vi "Zstack acquisition with modified signal input_final_3color.vi"() -> ()   [LabVIEW 2020]
uses:
  <vilib>/DAQmx/write.llb/DAQmx Write (Digital 1D Bool 1Chan 1Samp).vi
  <vilib>/DAQmx/write.llb/DAQmx Write (Analog 1D Wfm NChan NSamp).vi
  <vilib>/Analysis/polynomials.llb/Polynomial Plot (Range).vi
  <vilib>/Utility/file.llb/Read Delimited Spreadsheet (DBL).vi
  <vilib>/DAQmx/create/channels.llb/DAQmx Create Channel (AO-Voltage-Basic).vi
  <vilib>/DAQmx/create/channels.llb/DAQmx Create Channel (CO-Pulse Generation-Ticks).vi
  <vilib>/DAQmx/configure/timing.llb/DAQmx Timing (Sample Clock).vi
  <vilib>/DAQmx/configure/timing.llb/DAQmx Timing (Implicit).vi
  <vilib>/DAQmx/create/channels.llb/DAQmx Create Channel (DO-Digital Output).vi
  <vilib>/DAQmx/miscellaneous.llb/DAQmx Fill In Error Info.vi
  <vilib>/DAQmx/create/channels.llb/DAQmx Create Channel (CO-Pulse Generation-Frequency).vi
  <vilib>/Analysis/NI_AALPro.lvlib
  <resource>/objmgr/daqmx.rc
  <vilib>/measure/NI_MABase.lvlib
panel:
  out "number of samples written per channel":u32=1
  in  "Stop":bool
  out "LabVIEW generated Sawtooth input (blue) and Camera trigger (red)":waveform(dbl)[](graph)=[{"t0"=timestamp(0 s since 1904-01-01), "dt"=1.0, "Y"=array[3075 elements]}, {"t0"=timestamp(0 s since 1904-01-01), "dt"=0.001, "Y"=array[3075 elements]}, {"t0"=timestamp(0 s since 1904-01-01), "dt"=0.001, "Y"=array[3075 elements]}, {"t0"=timestamp(0 s since 1904-01-01), "dt"=0.001, "Y"=array[3075 elements]}]
  in  "stop 2":bool caption="stop"
  out "# Samples written per channel":u32=3075
  out "actual frequency":dbl=1000.0
  in  "stop":bool
  in  "File to read":path=path "C:/Users/Hannah/Downloads/newcalibration_voice coil input_25msflyback_3075datapoints.txt"
  in  "P(x)":dbl[](array[numeric])=[-0.285, 0.654, -0.163]
  out "polynomial plot":cluster{dbl[], "P(A)":dbl[]}(graph)
  out "Signal input to voice coil (blue)":dbl[](graph)=[-0.285, -0.284345508671835, -0.2836913439966493, -0.2830375059744429, -0.2823839946052158, -0.28173080988896804, -0.28107795182569956, -0.28042542041541035, -0.27977321565810054, -0.27912133755376994, -0.27846978610241874, -0.27781856130404675, -0.2771676631586541, -0.2765170916662408, -0.2758668468268068, -0.275216928640352, -0.27456733710687664, -0.27391807222638054, -0.2732691339988637, -0.2726205224243262, -0.271972237502768, -0.2713242792341891, -0.27067664761858956, -0.27002934265596923, -0.2693823643463283, -0.2687357126896666, -0.2680893876859843, -0.2674433893352812, -0.26679771763755744, -0.266152372592813, -0.2655073542010479, -0.26486266246226203, -0.2642182973764555, -0.2635742589436283, -0.2629305471637804, -0.26228716203691177, -0.2616441035630225, -0.26100137174211246, -0.2603589665741818, -0.2597168880592304, -0.2590751361972583, -0.2584337109882655, -0.25779261243225204, -0.25715184052921786, -0.256511395279163, -0.2558712766820875, -0.25523148473799123, -0.25459201944687426, -0.2539528808087366, -0.2533140688235783, -0.2526755834913993, -0.25203742481219954, -0.2513995927859791, -0.25076208741273803, -0.2501249086924762, -0.24948805662519374, -0.24885153121089054, -0.24821533244956667, -0.24757946034122208, -0.2469439148858568, -0.24630869608347083, -0.24567380393406418, -0.2450392384376368, -0.24440499959418877, -0.24377108740372, -0.24313750186623057, -0.24250424298172044, -0.2418713107501896, -0.2412387051716381, -0.24060642624606587, -0.23997447397347293, -0.23934284835385933, -0.23871154938722505, -0.23808057707357003, -0.23744993141289436, -0.23681961240519797, -0.2361896200504809, -0.2355599543487431, -0.23493061529998463, -0.23430160290420549, -0.23367291716140562, -0.23304455807158508, -0.23241652563474383, -0.23178881985088187, -0.23116144071999925, -0.23053438824209593, -0.2299076624171719, -0.22928126324522718, -0.22865519072626178, -0.22802944486027565, -0.22740402564726886, -0.22677893308724137, -0.22615416718019318, -0.2255297279261243, -0.22490561532503472, -0.22428182937692445, -0.22365837008179348, -0.22303523743964182, -0.22241243145046946, -0.2217899521142764, -0.22116779943106268, -0.2205459734008282, -0.21992447402357307, -0.21930330129929726, -0.21868245522800073, -0.21806193580968353, -0.2174417430443456, -0.216821876931987, -0.2162023374726077, -0.21558312466620771, -0.21496423851278704, -0.21434567901234564, -0.2137274461648836, -0.2131095399704008, -0.21249196042889734, -0.21187470754037319, -0.2112577813048283, -0.21064118172226276, -0.21002490879267655, -0.2094089625160696, -0.20879334289244195, -0.20817804992179365, -0.20756308360412462, -0.2069484439394349, -0.2063341309277245, -0.20572014456899337, -0.20510648486324162, -0.20449315181046912, -0.20388014541067592, -0.20326746566386203, -0.20265511257002744, -0.2020430861291722, -0.20143138634129623, -0.20082001320639958, -0.2002089667244822, -0.19959824689554417, -0.19898785371958544, -0.19837778719660598, -0.19776804732660586, -0.19715863410958503, -0.19654954754554352, -0.1959407876344813, -0.1953323543763984, -0.1947242477712948, -0.19411646781917047, -0.1935090145200255, -0.1929018878738598, -0.19229508788067345, -0.19168861454046637, -0.19108246785323857, -0.19047664781899015, -0.18987115443772096, -0.18926598770943112, -0.18866114763412056, -0.18805663421178936, -0.1874524474424374, -0.1868485873260648, -0.18624505386267143, -0.18564184705225745, -0.18503896689482274, -0.18443641339036732, -0.18383418653889122, -0.1832322863403944, -0.18263071279487691, -0.18202946590233876, -0.18142854566277988, -0.18082795207620028, -0.1802276851426, -0.17962774486197908, -0.17902813123433742, -0.17842884425967506, -0.17782988393799204, -0.17723125026928827, -0.17663294325356382, -0.1760349628908187, -0.1754373091810529, -0.17483998212426638, -0.17424298172045916, -0.17364630796963126, -0.17304996087178265, -0.17245394042691337, -0.1718582466350234, -0.1712628794961127, -0.17066783901018132, -0.17007312517722922, -0.1694787379972565, -0.16888467747026303, -0.16829094359624888, -0.167697536375214, -0.1671044558071585, -0.16651170189208225, -0.1659192746299853, -0.1653271740208677, -0.16473540006472936, -0.16414395276157034, -0.16355283211139066, -0.16296203811419024, -0.16237157076996914, -0.16178143007872733, -0.16119161604046486, -0.1606021286551817, -0.16001296792287784, -0.15942413384355322, -0.15883562641720797, -0.15824744564384202, -0.15765959152345535, -0.157072064056048, -0.15648486324161998, -0.15589798908017125, -0.1553114415717018, -0.15472522071621167, -0.15413932651370088, -0.15355375896416934, -0.15296851806761713, -0.15238360382404423, -0.15179901623345066, -0.15121475529583633, -0.15063082101120134, -0.15004721337954569, -0.1494639324008693, -0.14888097807517225, -0.14829835040245445, -0.14771604938271604, -0.14713407501595688, -0.14655242730217702, -0.1459711062413765, -0.14539011183355524, -0.14480944407871332, -0.1442291029768507, -0.1436490885279674, -0.14306940073206337, -0.14249003958913864, -0.14191100509919327, -0.14133229726222715, -0.1407539160782404, -0.14017586154723288, -0.1395981336692047, -0.13902073244415583, -0.13844365787208626, -0.13786690995299603, -0.13729048868688504, -0.1367143940737534, -0.13613862611360106, -0.13556318480642804, -0.1349880701522343, -0.13441328215101986, -0.13383882080278475, -0.1332646861075289, -0.1326908780652524, -0.1321173966759552, -0.1315442419396373, -0.1309714138562987, -0.13039891242593943, -0.12982673764855943, -0.12925488952415876, -0.1286833680527374, -0.12811217323429533, -0.12754130506883257, -0.12697076355634912, -0.12640054869684497, -0.1258306604903201, -0.1252610989367746, -0.12469186403620838, -0.12412295578862143, -0.12355437419401383, -0.12298611925238548, -0.12241819096373646, -0.1218505893280668, -0.12128331434537637, -0.1207163660156653, -0.1201497443389335, -0.119583449315181, -0.11901748094440787, -0.11845183922661395, -0.11788652416179943, -0.11732153574996412, -0.1167568739911082, -0.11619253888523154, -0.11562853043233423, -0.11506484863241617, -0.11450149348547742, -0.11393846499151802, -0.11337576315053788, -0.11281338796253709, -0.11225133942751558, -0.11168961754547335, -0.11112822231641048, -0.11056715374032686, -0.1100064118172226, -0.10944599654709763, -0.10888590792995195, -0.10832614596578558, -0.10776671065459853, -0.10720760199639076, -0.1066488199911623, -0.10609036463891316, -0.10553223593964331, -0.10497443389335279, -0.10441695850004157, -0.10385980975970963, -0.10330298767235702, -0.10274649223798371, -0.10219032345658968, -0.10163448132817499, -0.1010789658527396, -0.1005237770302835, -0.09996891486080672, -0.09941437934430924, -0.09886017048079107, -0.0983062882702522, -0.09775273271269264, -0.0971995038081124, -0.09664660155651142, -0.0960940259578898, -0.09554177701224745, -0.0949898547195844, -0.09443825907990072, -0.09388699009319626, -0.09333604775947113, -0.09278543207872533, -0.09223514305095881, -0.09168518067617165, -0.09113554495436374, -0.09058623588553519, -0.09003725346968586, -0.08948859770681591, -0.08894026859692525, -0.08839226614001383, -0.0878445903360818, -0.08729724118512902, -0.0867502186871556, -0.08620352284216146, -0.08565715365014659, -0.08511111111111108, -0.08456539522505482, -0.08402000599197795, -0.08347494341188033, -0.08293020748476201, -0.082385798210623, -0.08184171558946332, -0.08129795962128292, -0.08075453030608179, -0.08021142764386005, -0.07966865163461759, -0.0791262022783544, -0.07858407957507055, -0.07804228352476594, -0.07750081412744073, -0.07695967138309479, -0.07641885529172815, -0.07587836585334079, -0.07533820306793276, -0.07479836693550404, -0.07425885745605462, -0.07371967462958451, -0.0731808184560937, -0.0726422889355822, -0.07210408606805, -0.07156620985349715, -0.0710286602919235, -0.07049143738332925, -0.06995454112771426, -0.06941797152507859, -0.06888172857542227, -0.06834581227874517, -0.0678102226350474, -0.06727495964432897, -0.06674002330658982, -0.06620541362183, -0.06567113059004948, -0.06513717421124829, -0.06460354448542632, -0.06407024141258374, -0.06353726499272042, -0.06300461522583639, -0.062472292111931726, -0.06194029565100631, -0.061408625843060255, -0.06087728268809345, -0.060346266186105973, -0.05981557633709783, -0.05928521314106894, -0.05875517659801943, -0.05822546670794915, -0.05769608347085822, -0.057167026886746575, -0.05663829695561426, -0.05610989367746122, -0.05558181705228746, -0.05505406708009308, -0.05452664376087796, -0.053999547094642164, -0.053472777081385675, -0.052946333721108435, -0.05242021701381058, -0.05189442695949201, -0.05136896355815271, -0.05084382680979274, -0.05031901671441208, -0.04979453327201072, -0.04927037648258867, -0.04874654634614592, -0.048223042862682475, -0.047699866032198335, -0.0471770158546935, -0.04665449233016797, -0.04613229545862174, -0.04561042524005482, -0.04508888167446723, -0.044567664761858916, -0.044046774502229935, -0.04352621089558023, -0.04300597394190983, -0.04248606364121876, -0.04196647999350697, -0.04144722299877451, -0.04092829265702133, -0.04040968896824751, -0.039891411932452936, -0.03937346154963772, -0.03885583781980173, -0.0383385407429451, -0.0378215703190678, -0.03730492654816975, -0.03678860943025106, -0.036272618965311615, -0.035756955153351505, -0.03524161799437073, -0.0347266074883692, -0.03421192363534703, -0.03369756643530414, -0.03318353588824058, -0.03266983199415624, -0.032156454753051344, -0.03164340416492567, -0.031130680229779273, -0.030618282947612263, -0.030106212318424475, -0.029594468342216074, -0.02908305101898695, -0.028571960348737047, -0.028061196331466587, -0.027550758967175293, -0.027040648255863442, -0.026530864197530812, -0.026021406792177515, -0.02551227603980355, -0.02500347194040886, -0.02449499449399345, -0.02398684370055737, -0.023479019560100622, -0.02297152207262315, -0.022464351238125013, -0.021957507056606096, -0.021450989528066566, -0.020944798652506313, -0.020438934429925393, -0.01993339686032375, -0.019428185943701437, -0.018923301680058457, -0.0184187440693947, -0.01791451311171033, -0.01741060880700518, -0.01690703115527936, -0.016403780156532932, -0.01590085581076567, -0.015398258117977848, -0.014895987078169193, -0.014394042691339926, -0.01389242495748999, -0.013391133876619332, -0.012890169448728006, -0.012389531673815901, -0.011889220551883184, -0.011389236082929743, -0.01088957826695558, -0.010390247103960804, -0.009891242593945249, -0.009392564736909081, -0.008894213532852135, -0.008396188981774577, -0.00789849108367624, -0.007401119838557235, -0.0069040752464175625, -0.006407357307257167, -0.005910966021076103, -0.005414901387874316, -0.004919163407651805, -0.004423752080408738, -0.003928667406144837, -0.003433909384860323, -0.002939478016555086, -0.0024453733012291257, -0.0019515952388824975, -0.0014581438295152016, -0.0009650190731271269, -0.00047222096971838434, 2.0250480710970464e-05, 0.0005123952781611041, 0.00100421342263185, 0.0014957049141233747, 0.0019868697526356227, 0.0024777079381684275, 0.002968219470722011, 0.0034584043502962625, 0.003948262576891293, 0.00443779415050688, 0.004926999071143245, 0.005415877338800279, 0.00590442895347798, 0.006392653915176516, 0.0068805522238956085, 0.007368123879635424, 0.007855368882395908, 0.008342287232177115, 0.0088288789289791, 0.009315143972801698, 0.009801082363644964, 0.010286694101508898, 0.01077197918639361, 0.01125693761829899, 0.011741569397225093, 0.012225874523171809, 0.012709852996139304, 0.013193504816127466, 0.013676829983136352, 0.014159828497165905, 0.01464250035821607, 0.015124845566287015, 0.015606864121378683, 0.01608855602349102, 0.016569921272624022, 0.017050959868777693, 0.017531671811952143, 0.018012057102147205, 0.018492115739363046, 0.0189718477235995, 0.019451253054856676, 0.019930331733134576, 0.02040908375843309, 0.020887509130752435, 0.02136560785009234, 0.02184337991645302, 0.02232082532983437, 0.02279794409023639, 0.023274736197659185, 0.023751201652102594, 0.024227340453566726, 0.024703152602051526, 0.025178638097557104, 0.025653796940083295, 0.026128629129630154, 0.026603134666197792, 0.027077313549786042, 0.02755116578039507, 0.02802469135802471, 0.028497890282675076, 0.028970762554346163, 0.02944330817303792, 0.029915527138750453, 0.030387419451483544, 0.030858985111237414, 0.03133022411801195, 0.031801136471807157, 0.03227172217262314, 0.03274198122045974, 0.03321191361531706, 0.033681519357195044, 0.034150798446093755, 0.03461975088201319, 0.03508837666495329, 0.03555667579491412, 0.036024648271895554, 0.036492294095897715, 0.0369596132669206, 0.037426605784964206, 0.03789327165002848, 0.03835961086211337, 0.038825623421219035, 0.039291309327345425, 0.03975666858049248, 0.04022170118066015, 0.0406864071278486, 0.04115078642205772, 0.041614839063287556, 0.042078565051538064, 0.04254196438680924, 0.04300503706910114, 0.043467783098413704, 0.043930202474747104, 0.04439229519810106, 0.04485406126847569, 0.04531550068587109, 0.04577661345028711, 0.04623739956172396, 0.046697859020181365, 0.04715799182565955, 0.047617797978158405, 0.04807727747767787, 0.04853643032421817, 0.048995256517779084, 0.04945375605836072, 0.04991192894596297, 0.050369775180585996, 0.0508272947622298, 0.05128448769089411, 0.05174135396657925, 0.05219789358928495, 0.05265410655901154, 0.05310999287575868, 0.05356555253952655, 0.05402078555031514, 0.054475691908124346, 0.054930271612954384, 0.05538452466480498, 0.05583845106367635, 0.05629205080956834, 0.05674532390248105, 0.05719827034241459, 0.05765089012936864, 0.05810318326334346, 0.05855514974433895, 0.05900678957235517, 0.05945810274739205, 0.059909089269449656, 0.060359749138527985, 0.060810082354626926, 0.06126008891774659, 0.06170976882788698, 0.06215912208504809, 0.06260814868922976, 0.06305684864043226, 0.06350522193865543, 0.06395326858389927, 0.06440098857616383, 0.064848381915449, 0.06529544860175496, 0.06574218863508158, 0.06618860201542892, 0.06663468874279693, 0.06708044881718556, 0.06752588223859501, 0.06797098900702508, 0.06841576912247588, 0.06886022258494734, 0.06930434939443952, 0.06974814955095238, 0.0701916230544859, 0.07063476990504025, 0.07107759010261516, 0.0715200836472108, 0.07196225053882715, 0.07240409077746413, 0.07284560436312199, 0.07328679129580035, 0.07372765157549949, 0.0741681852022193, 0.07460839217595977, 0.07504827249672097, 0.07548782616450289, 0.07592705317930548, 0.07636595354112874, 0.07680452724997272, 0.07724277430583737, 0.0776806947087228, 0.07811828845862884, 0.07855555555555555, 0.07899249599950303, 0.07942910979047119, 0.07986539692846006, 0.08030135741346961, 0.08073699124549977, 0.0811722984245507, 0.08160727895062231, 0.08204193282371469, 0.08247626004382763, 0.08291026061096135, 0.08334393452511574, 0.08377728178629085, 0.08421030239448662, 0.08464299634970307, 0.08507536365194024, 0.08550740430119813, 0.08593911829747669, 0.08637050564077597, 0.08680156633109587, 0.08723230036843654, 0.08766270775279789, 0.08809278848417995, 0.08852254256258263, 0.08895196998800603, 0.08938107076045021, 0.089809844879915, 0.09023829234640052, 0.0906664131599067, 0.0910942073204336, 0.09152167482798113, 0.09194881568254948, 0.0923756298841385, 0.09280211743274808, 0.09322827832837849, 0.09365411257102946, 0.09407962016070132, 0.09450480109739373, 0.09492965538110687, 0.09535418301184073, 0.0957783839895952, 0.09620225831437051, 0.09662580598616638, 0.09704902700498302, 0.09747192137082028, 0.09789448908367826, 0.09831673014355707, 0.09873864455045639, 0.09916023230437648, 0.09958149340531725, 0.10000242785327873, 0.10042303564826088, 0.10084331679026376, 0.10126327127928736, 0.10168289911533157, 0.1021022002983965, 0.10252117482848216, 0.10293982270558855, 0.10335814392971548, 0.10377613850086326, 0.1041938064190317, 0.1046111476842208, 0.10502816229643064, 0.10544485025566108, 0.1058612115619123, 0.1062772462151842, 0.10669295421547681, 0.10710833556279009, 0.10752339025712399, 0.10793811829847871, 0.10835251968685405, 0.10876659442225012, 0.10918034250466685, 0.1095937639341043, 0.11000685871056248, 0.11041962683404127, 0.11083206830454084, 0.11124418312206102, 0.11165597128660193, 0.11206743279816361, 0.11247856765674591, 0.11288937586234893, 0.11329985741497256, 0.11371001231461697, 0.114119840561282, 0.11452934215496785, 0.11493851709567426, 0.11534736538340146, 0.11575588701814932, 0.11616408199991785, 0.11657195032870715, 0.11697949200451707, 0.11738670702734771, 0.11779359539719908, 0.11820015711407106, 0.11860639217796382, 0.11901230058887718, 0.11941788234681133, 0.11982313745176615, 0.12022806590374158, 0.12063266770273778, 0.12103694284875471, 0.12144089134179231, 0.12184451318185052, 0.12224780836892951, 0.12265077690302917, 0.12305341878414955, 0.12345573401229065, 0.12385772258745231, 0.12425938450963481, 0.12466071977883791, 0.1250617283950618, 0.12546241035830635, 0.12586276566857152, 0.12626279432585746, 0.12666249633016402, 0.12706187168149136, 0.1274609203798393, 0.12785964242520803, 0.12825803781759737, 0.1286561065570075, 0.12905384864343833, 0.12945126407688973, 0.1298483528573619, 0.1302451149848547, 0.13064155045936832, 0.1310376592809026, 0.1314334414494575, 0.13182889696503314, 0.13222402582762943, 0.1326188280372465, 0.1330133035938842, 0.1334074524975426, 0.13380127474822168, 0.13419477034592148, 0.13458793929064206, 0.1349807815823832, 0.1353732972211451, 0.13576548620692763, 0.136157348539731, 0.13654888421955497, 0.1369400932463996, 0.13733097562026497, 0.13772153134115095, 0.13811176040905782, 0.13850166282398518, 0.13889123858593333, 0.1392804876949021, 0.13966941015089163, 0.14005800595390194, 0.14044627510393282, 0.1408342176009844, 0.14122183344505668, 0.14160912263614966, 0.14199608517426343, 0.14238272105939775, 0.14276903029155286, 0.14315501287072857, 0.14354066879692506, 0.14392599807014222, 0.1443110006903801, 0.1446956766576386, 0.14508002597191788, 0.14546404863321782, 0.1458477446415385, 0.14623111399687982, 0.14661415669924177, 0.14699687274862455, 0.14737926214502794, 0.14776132488845206, 0.1481430609788969, 0.1485244704163623, 0.14890555320084853, 0.14928630933235543, 0.149666738810883, 0.15004684163643123, 0.15042661780900024, 0.15080606732858992, 0.15118519019520027, 0.15156398640883134, 0.15194245596948303, 0.1523205988771555, 0.15269841513184862, 0.15307590473356236, 0.153453067682297, 0.15382990397805213, 0.1542064136208281, 0.15458259661062473, 0.15495845294744193, 0.15533398263127995, 0.15570918566213865, 0.15608406204001807, 0.15645861176491815, 0.15683283483683885, 0.15720673125578033, 0.15758030102174247, 0.1579535441347254, 0.15832646059472888, 0.1586990504017532, 0.15907131355579807, 0.15944325005686372, 0.1598148599049501, 0.16018614310005702, 0.16055709964218473, 0.16092772953133316, 0.16129803276750232, 0.16166800935069214, 0.16203765928090252, 0.16240698255813374, 0.16277597918238562, 0.16314464915365823, 0.16351299247195145, 0.16388100913726544, 0.16424869914960005, 0.16461606250895544, 0.16498309921533155, 0.16534980926872822, 0.16571619266914567, 0.16608224941658378, 0.16644797951104262, 0.16681338295252218, 0.16717845974102236, 0.16754320987654325, 0.16790763335908487, 0.16827173018864716, 0.16863550036523012, 0.1689989438888338, 0.16936206075945814, 0.16972485097710327, 0.17008731454176906, 0.17044945145345547, 0.17081126171216265, 0.17117274531789045, 0.17153390227063908, 0.17189473257040833, 0.17225523621719824, 0.17261541321100887, 0.17297526355184012, 0.17333478723969226, 0.1736939842745649, 0.1740528546564583, 0.17441139838537234, 0.17476961546130715, 0.17512750588426274, 0.17548506965423888, 0.17584230677123575, 0.17619921723525328, 0.17655580104629154, 0.17691205820435063, 0.17726798870943017, 0.1776235925615306, 0.17797886976065153, 0.1783338203067933, 0.17868844419995572, 0.17904274144013888, 0.17939671202734264, 0.1797503559615672, 0.18010367324281246, 0.18045666387107834, 0.18080932784636494, 0.18116166516867216, 0.1815136758380002, 0.18186535985434893, 0.18221671721771826, 0.18256774792810837, 0.18291845198551904, 0.18326882938995054, 0.1836188801414027, 0.18396860423987554, 0.18431800168536905, 0.18466707247788333, 0.18501581661741828, 0.1853642341039739, 0.18571232493755024, 0.1860600891181472, 0.18640752664576493, 0.18675463752040333, 0.18710142174206246, 0.18744787931074225, 0.18779401022644265, 0.1881398144891639, 0.18848529209890574, 0.18883044305566837, 0.18917526735945162, 0.18951976501025553, 0.18986393600808021, 0.19020778035292546, 0.1905512980447916, 0.19089448908367834, 0.19123735346958576, 0.19157989120251384, 0.19192210228246265, 0.19226398670943223, 0.19260554448342238, 0.1929467756044333, 0.19328768007246488, 0.19362825788751714, 0.19396850904959018, 0.19430843355868382, 0.19464803141479825, 0.19498730261793323, 0.19532624716808905, 0.19566486506526554, 0.19600315630946263, 0.19634112090068057, 0.196678758838919, 0.19701607012417827, 0.1973530547564582, 0.19768971273575886, 0.19802604406208013, 0.19836204873542213, 0.19869772675578484, 0.19903307812316823, 0.1993681028375724, 0.1997028008989971, 0.2000371723074426, 0.20037121706290878, 0.20070493516539567, 0.20103832661490328, 0.20137139141143146, 0.20170412955498046, 0.20203654104555008, 0.20236862588314047, 0.20270038406775148, 0.20303181559938321, 0.20336292047803567, 0.20369369870370874, 0.20402415027640258, 0.2043542751961171, 0.20468407346285228, 0.20501354507660818, 0.2053426900373848, 0.2056715083451821, 0.20600000000000002]
  out "Error out":errorcluster
  in  "Disable Axis":bool
  in  "Z step size (um)":dbl=0.2
  out "Number of Slices":dbl=400.0
  in  "Input will be multiplied by 5":dbl=80.0
  in  "Acquire Z Stack?":bool=TRUE
  out "GetFirmwareVersion 2":string="3.03\r"
  out "Connected":bool=TRUE
  in  "SPIIPLUSCOM660Lib.IAsyncChannel":refnum<k7>
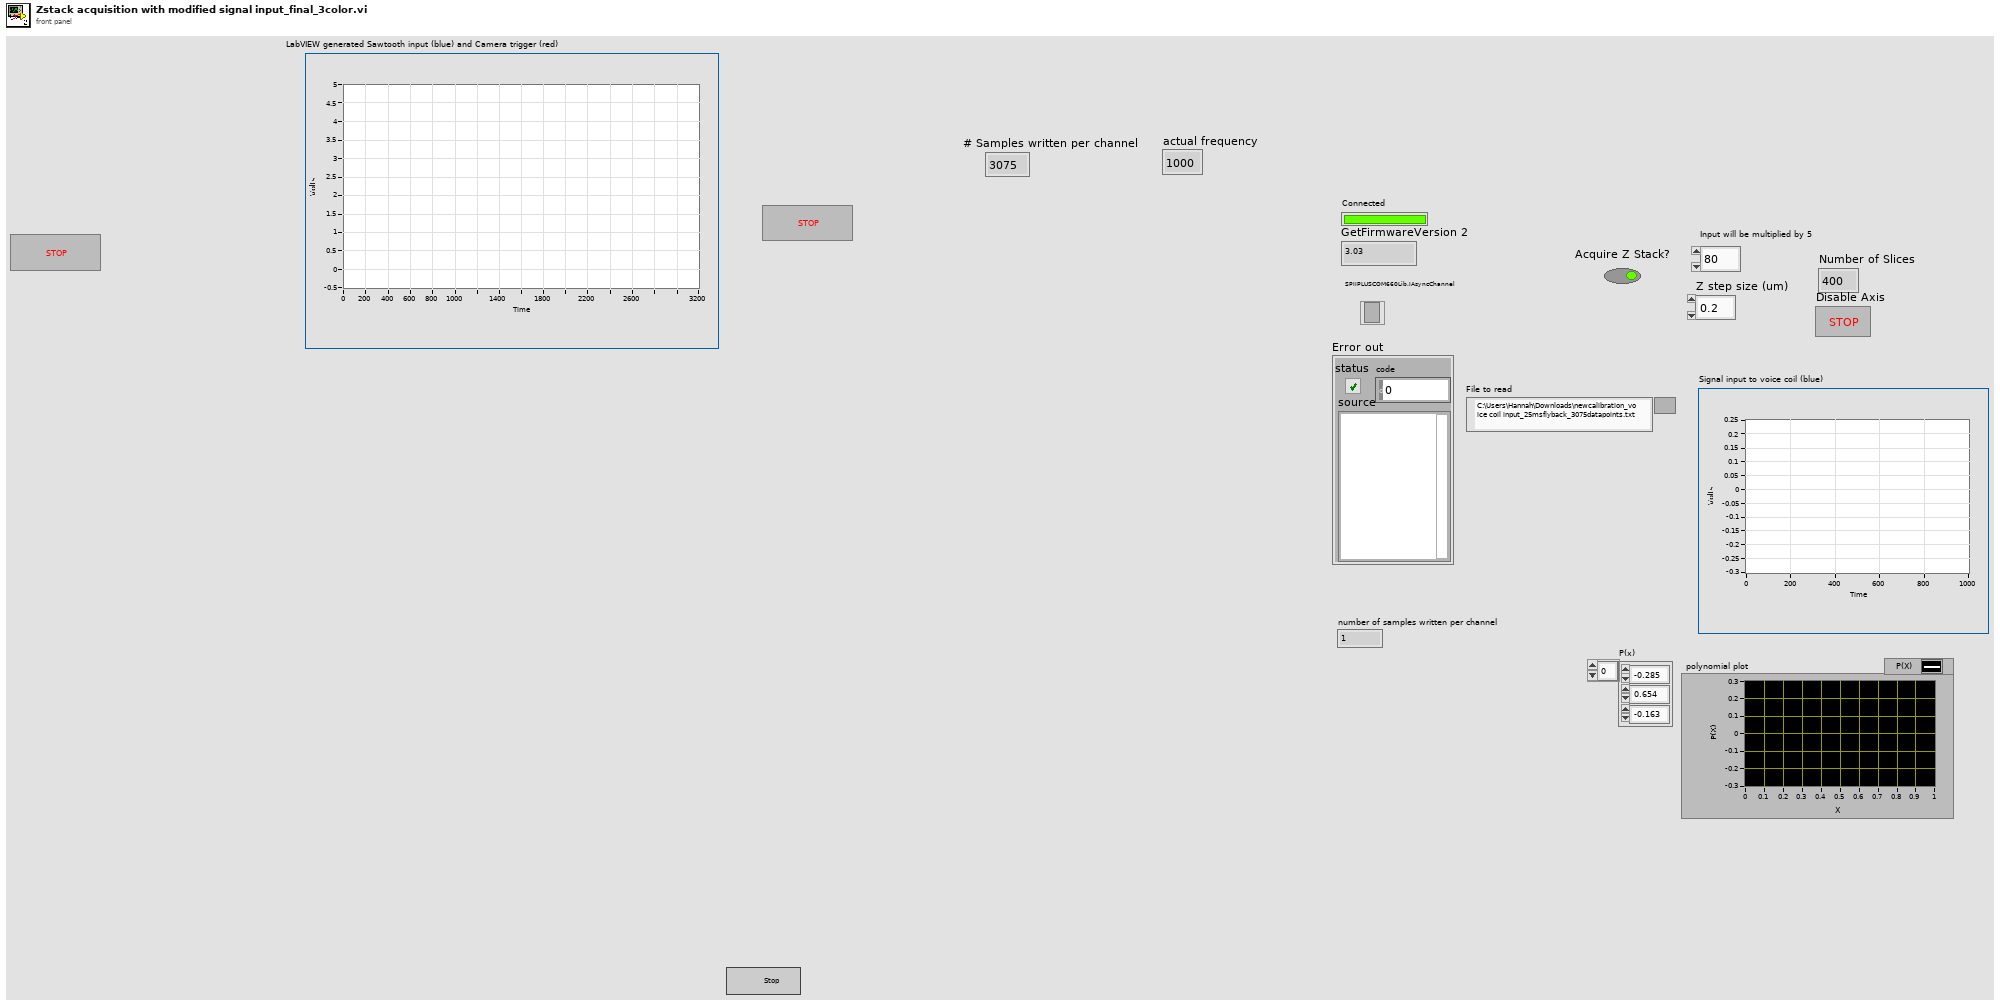
[diagram p1: front panel]
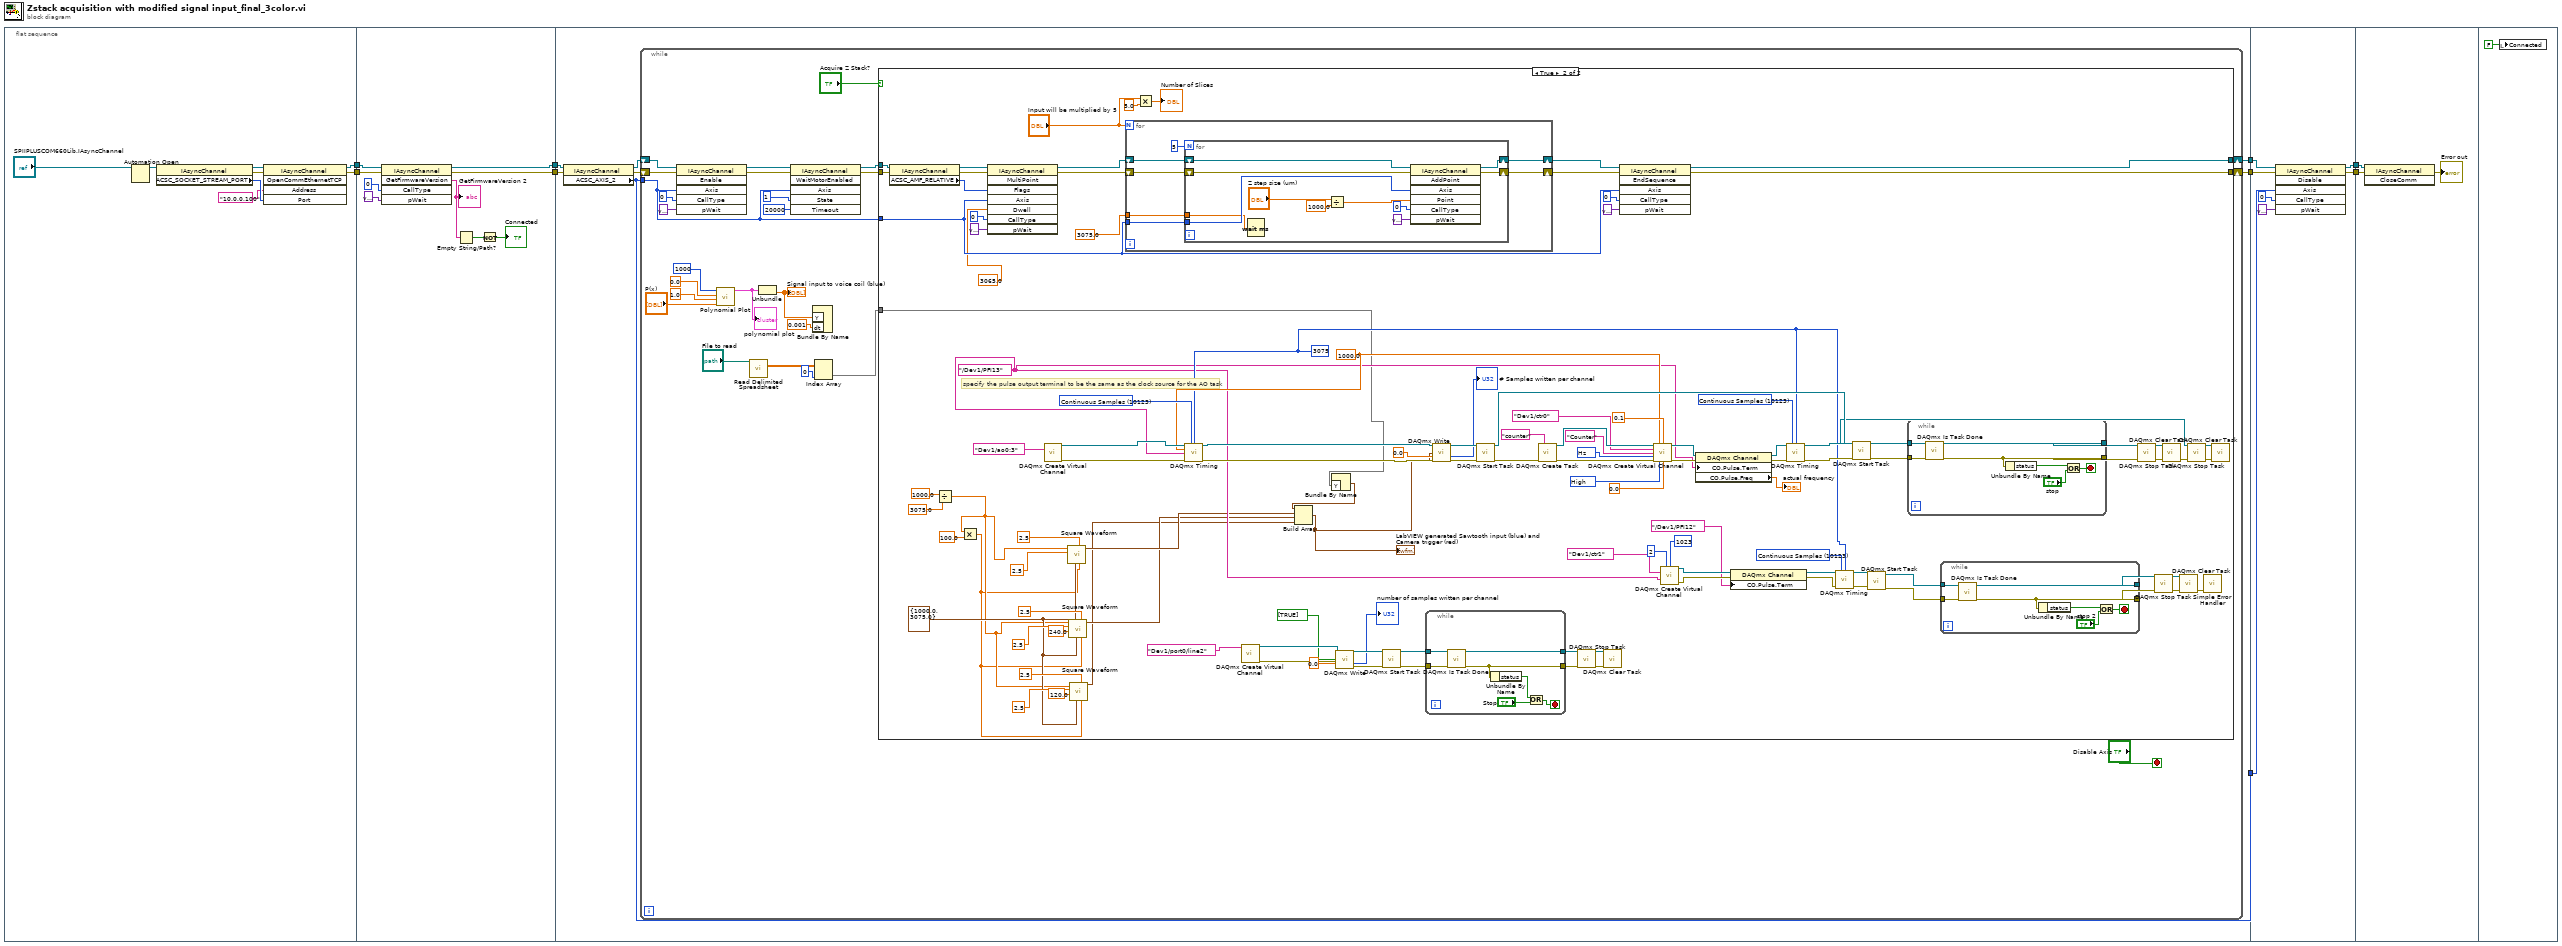
[diagram p0: block diagram]
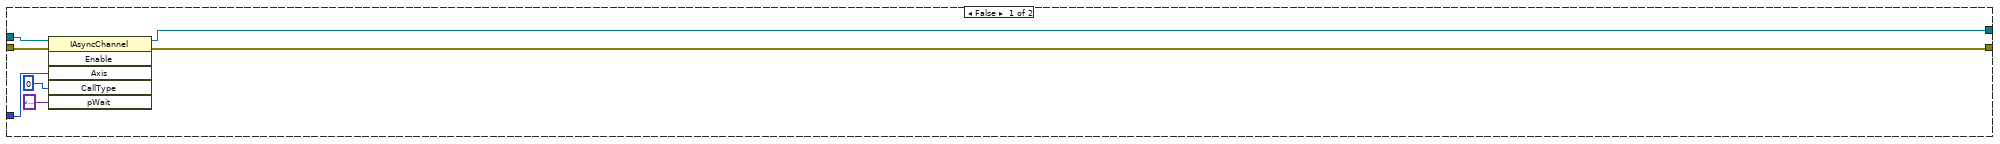
[diagram p2: hidden frame]
diagram:
  n1 = flat-sequence {
    tunnel: [w12] -> w9
    tunnel: [w11] -> w8
    tunnel: w9 -> [w22]
    tunnel: w8 -> [w21]
    tunnel: [w19] -> w7
    tunnel: [w18] -> w6
    tunnel: w7 -> [w31]
    tunnel: w6 -> [w30]
    tunnel: [w33] -> w5
    tunnel: [w32] -> w4
    tunnel: [w29] -> w3
    tunnel: w5 -> [w226]
    tunnel: w4 -> [w225]
    tunnel: [w224] -> w2
    tunnel: [w223] -> w1
    tunnel: w3 -> [w222]
    tunnel: w2 -> [w228]
    tunnel: w1 -> [w227]
    frame #0 {
      n2 = Automation Open(Automation Refnum="SPIIPLUSCOM660Lib.IAsyncChannel") -> (Automation Refnum=w17:refnum<k7>)  [unwired: 3 in, 1 out]
      n3 = property class="IAsyncChannel"(reference=w17) -> (reference out=w16:refnum<k7>, error out=w10:errorcluster, "ACSC_SOCKET_STREAM_PORT"=w14:i32)  [unwired: 1 in]
      n4 = invoke class="IAsyncChannel" method="OpenCommEthernetTCP"(reference=w16, error in=w10, "Address"="10.0.0.100", "Port"=w14) -> (reference out=w12:refnum<k7>, error out=w11:errorcluster)  [unwired: 1 in, 3 out]
    }
    frame #1 {
      n5 = invoke class="IAsyncChannel" method="GetFirmwareVersion"(reference=w22, error in=w21, "CallType"=u64 0, "pWait"=variant) -> (reference out=w19:refnum<k7>, error out=w18:errorcluster, "GetFirmwareVersion"=w24:string)  [unwired: 1 in, 2 out]
      "GetFirmwareVersion 2" <- w24
      n6 = Empty String/Path?(string/path=w24) -> (empty?=w23:bool)
      n7 = Not(x=w23) -> (.not. x?=→"Connected":bool)
    }
    frame #2 {
      n8 = property class="IAsyncChannel"(reference=w31, error in=w30) -> (reference out=w28:refnum<k7>, error out=w27:errorcluster, "ACSC_AXIS_2"=w29:i32)
      n9 = while {
        shift-right: [w59] -> w33
        shift-left: w28 -> [w51]
        shift-right: [w58] -> w32
        shift-left: w27 -> [w50]
        tunnel: w29 -> [w47]
        stop <- "Disable Axis" stop-if-true
        n10 = invoke class="IAsyncChannel" method="Enable"(reference=w51, error in=w50, "Axis"=w47, "CallType"=u64 0, "pWait"=variant) -> (reference out=w55:refnum<k7>, error out=w54:errorcluster)  [unwired: 1 in, 4 out]
        n11 = call-poly <vilib>:"Polynomial Plot.vi"("P(x)"="P(x)", "end"=1.0, "start"=0.0, "samples"=1000) -> ("polynomial plot"=w43:cluster{"Ramp Pattern":dbl[], "P(A)":dbl[]})  [unwired: 6 in, 1 out]
        "polynomial plot" <- w43
        n12 = call-poly <vilib>:"Read Delimited Spreadsheet.vi"("file path (dialog if empty)"="File to read") -> ("all rows"=w36:dbl[][])  [unwired: 9 in, 5 out]
        n13 = Unbundle(w43) -> ("P(A)"=w38:dbl[])  [unwired: 1 out]
        "Signal input to voice coil (blue)" <- w38
        n14 = invoke class="IAsyncChannel" method="WaitMotorEnabled"(reference=w55, error in=w54, "Axis"=w47, "State"=1, "Timeout"=20000) -> (reference out=w46:refnum<k7>, error out=w45:errorcluster)  [unwired: 1 in, 4 out]
        n15 = Bundle By Name("Y"=w38, "dt"=0.001) -> ()  [unwired: 1 in, 1 out]
        n16 = Index Array(array=w36, index (col)=0 ("disabled index (col)")) -> (element=w34:dbl[])  [unwired: 1 in]
        n17 = case shown="True" "Acquire Z Stack?" {
          tunnel: w46 -> [w66 w168]
          tunnel: w45 -> [w65 w169]
          tunnel: [w64 w166] -> w59
          tunnel: [w63 w167] -> w58
          tunnel: w47 -> [w62 w165]
          tunnel: w34 -> [_ w86]
          frame False {
            n18 = invoke class="IAsyncChannel" method="Enable"(reference=w66, error in=w65, "Axis"=w62, "CallType"=u64 0, "pWait"=variant) -> (reference out=w64:refnum<k7>, error out=w63:errorcluster)  [unwired: 1 in, 4 out]
          }
          frame True {
            w71 = cluster{"Fs":dbl, "#s":dbl} {"Fs"=1000.0, "#s"=3075.0} ("sampling info")
            w102 = 3075 ("samples per channel")
            w105 = 10123 items=["Finite Samples"=10178, "Continuous Samples"=10123, "Hardware Timed Single Point"=12522] ("sample mode")
            w131 = 10192 items=["High"=10192, "Low"=10214] ("idle state")
            w132 = 10373 items=["Hz"=10373] ("units")
            w101 = tag "/Dev1/PFI13" ("CO.Pulse.Term")
            w119 = 10123 items=["Finite Samples"=10178, "Continuous Samples"=10123, "Hardware Timed Single Point"=12522] ("sample mode")
            w115 = 1000.0 ("rate")
            w157 = 10123 items=["Finite Samples"=10178, "Continuous Samples"=10123, "Hardware Timed Single Point"=12522] ("sample mode")
            # "specify the pulse output terminal to be the same as the clock source for the AO task"
            n19 = property class="IAsyncChannel"(reference=w168, error in=w169) -> (reference out=w178:refnum<k7>, error out=w177:errorcluster, "ACSC_AMF_RELATIVE"=w174:i32)
            n20 = Divide(x=1000.0, y=3075.0) -> (x/y=w69:dbl)
            n21 = Multiply(x=w69, y=100.0) -> (x*y=w68:dbl)
            n22 = invoke class="IAsyncChannel" method="MultiPoint"(reference=w178, error in=w177, "Flags"=w174, "Axis"=w165, "Dwell"=3065.0, "CallType"=u64 0, "pWait"=variant) -> (reference out=w173:refnum<k7>, error out=w172:errorcluster)  [unwired: 1 in, 6 out]
            n23 = call-poly <vilib>:"DAQmx Create Virtual Channel.vi"("physical channels"=tag "Dev1/ao0:3") -> ("task out"=w159:refnum<k21>, "error out"=w158:errorcluster)  [unwired: 13 in]
            n24 = call <vilib>:"Square Waveform.vi"("duty cycle (%)"=w68, "offset"=2.5, "sampling info"=w71, "amplitude"=2.5 ("Amplitude for laser 1 (Max value 2.5)"), "frequency"=w69) -> ("signal out"=w99:waveform(dbl))  [unwired: 5 in, 1 out]
            n25 = call <vilib>:"Square Waveform.vi"("duty cycle (%)"=w68, "offset"=2.5, "sampling info"=w71, "phase"=240.0, "amplitude"=2.5 ("Amplitude for laser 1 (Max value 2.5)"), "frequency"=w69) -> ("signal out"=w95:waveform(dbl))  [unwired: 4 in, 1 out]
            n26 = call <vilib>:"Square Waveform.vi"("duty cycle (%)"=w68, "offset"=2.5, "sampling info"=w71, "phase"=120.0, "amplitude"=2.5 ("Amplitude for laser 1 (Max value 2.5)"), "frequency"=w69) -> ("signal out"=w92:waveform(dbl))  [unwired: 4 in, 1 out]
            n27 = for {
              N: "Input will be multiplied by 5" -> [_]
              tunnel: w165 -> [w204]
              tunnel: 3075.0 ("Dwell") -> [w203]
              shift-right: [w206] -> w171
              shift-left: w173 -> [w208]
              shift-right: [w205] -> w170
              shift-left: w172 -> [w207]
              n28 = for {
                N: 5 -> [_]
                tunnel: w204 -> [w219]
                shift-right: [w214] -> w206
                shift-left: w208 -> [w218]
                shift-right: [w213] -> w205
                shift-left: w207 -> [w217]
                tunnel: w203 -> [w209]
                n29 = Wait (ms)(milliseconds to wait=w209) -> ()  [unwired: 1 out]
                n30 = Divide(x="Z step size (um)", y=1000.0) -> (x/y=w210:dbl)
                n31 = invoke class="IAsyncChannel" method="AddPoint"(reference=w218, error in=w217, "Axis"=w219, "Point"=w210, "CallType"=u64 0, "pWait"=variant) -> (reference out=w214:refnum<k7>, error out=w213:errorcluster)  [unwired: 1 in, 5 out]
              }
            }
            n32 = Multiply(x="Input will be multiplied by 5", y=5.0) -> (x*y=→"Number of Slices":dbl)
            n33 = call-poly <vilib>:"DAQmx Timing.vi"("task/channels in"=w159, "sample mode"=w157, "samples per channel"=w102, "rate"=w115, "source"=w101, "error in"=w158) -> ("task out"=w124:refnum<k21>, "error out"=w123:errorcluster)  [unwired: 8 in]
            n34 = call-poly <vilib>:"DAQmx Create Virtual Channel.vi"("lines"=tag "Dev1/port0/line2") -> ("task out"=w85:refnum<k21>, "error out"=w84:errorcluster)  [unwired: 13 in]
            n35 = Bundle By Name("Y"=w86) -> (w88:waveform(dbl))  [unwired: 1 in]
            n36 = Build Array(w88, w99, w95, w92) -> (w87:waveform(dbl)[])
            "LabVIEW generated Sawtooth input (blue) and Camera trigger (red)" <- w87
            n37 = call-poly <vilib>:"DAQmx Write.vi"("task/channels in"=w85, "data"=bool[] [TRUE], "timeout"=0.0, "error in"=w84) -> ("task out"=w83:refnum<k21>, "number of samples written per channel"=→"number of samples written per channel":u32, "error out"=w82:errorcluster)  [unwired: 9 in]
            n38 = call <vilib>:"DAQmx Start Task.vi"("task/channels in"=w83, "error in"=w82) -> ("task out"=w81:refnum<k21>, "error out"=w80:errorcluster)  [unwired: 12 in]
            n39 = while {
              tunnel: w81 -> [w187]
              tunnel: w80 -> [w186]
              tunnel: [w184] -> w76
              tunnel: [w185] -> w77
              stop <- w181 stop-if-true
              n40 = call <vilib>:"DAQmx Is Task Done.vi"("task/channels in"=w187, "error in"=w186) -> ("task out"=w185:refnum<k21>, "error out"=w184:errorcluster)  [unwired: 11 in, 1 out]
              n41 = Unbundle By Name(w184) -> ("status"=w183:bool)
              n42 = Or(x=w183, y="Stop") -> (x .or. y?=w181:bool)
            }
            n43 = call-poly <vilib>:"DAQmx Write.vi"("task/channels in"=w124, "data"=w87, "timeout"=0.0, "error in"=w123) -> ("task out"=w137:refnum<k21>, "number of samples written per channel"=→"# Samples written per channel":u32, "error out"=w136:errorcluster)  [unwired: 9 in]
            n44 = call <vilib>:"DAQmx Start Task.vi"("task/channels in"=w137, "error in"=w136) -> ("task out"=w130:refnum<k21>, "error out"=w129:errorcluster)  [unwired: 12 in]
            n45 = call <vilib>:"DAQmx Create Task.vi"("new task name"="counter", "error in"=w129) -> ("task out"=w152:refnum<k21>, "error out"=w150:errorcluster)  [unwired: 12 in]
            n46 = call <vilib>:"DAQmx Stop Task.vi"("task/channels in"=w77, "error in"=w76) -> ("task out"=w79:refnum<k21>, "error out"=w78:errorcluster)  [unwired: 12 in]
            n47 = call <vilib>:"DAQmx Clear Task.vi"("task in"=w79, "error in"=w78) -> ()  [unwired: 13 in, 1 out]
            n48 = invoke class="IAsyncChannel" method="EndSequence"(reference=w171, error in=w170, "Axis"=w165, "CallType"=u64 0, "pWait"=variant) -> (reference out=w166:refnum<k7>, error out=w167:errorcluster)  [unwired: 1 in, 4 out]
            n49 = call-poly <vilib>:"DAQmx Create Virtual Channel.vi"("task in"=w152, "frequency"=w115, "duty cycle"=0.1, "counter"=tag "Dev1/ctr0", "name to assign"="Counter", "units"=w132, "error in"=w150, "idle state"=w131, "initial delay"=0.0) -> ("task out"=w149:refnum<k21>, "error out"=w148:errorcluster)  [unwired: 5 in]
            n50 = call-poly <vilib>:"DAQmx Create Virtual Channel.vi"("high ticks"=u32 2, "low ticks"=u32 1023, "counter"=tag "Dev1/ctr1", "source of ticks"=w101) -> ("task out"=w114:refnum<k21>, "error out"=w113:errorcluster)  [unwired: 10 in]
            n51 = property class="DAQmx Channel"(reference=w149, error in=w148, "CO.Pulse.Term"=w101) -> (reference out=w145:refnum<k21>, error out=w146:errorcluster, "CO.Pulse.Freq"=→"actual frequency":dbl)
            n52 = property class="DAQmx Channel"(reference=w114, error in=w113, "CO.Pulse.Term"=tag "/Dev1/PFI12") -> (reference out=w107:refnum<k21>, error out=w106:errorcluster)
            n53 = call-poly <vilib>:"DAQmx Timing.vi"("task/channels in"=w145, "sample mode"=w119, "samples per channel"=w102, "error in"=w146) -> ("task out"=w155:refnum<k21>, "error out"=w154:errorcluster)  [unwired: 10 in]
            n54 = call-poly <vilib>:"DAQmx Timing.vi"("task/channels in"=w107, "sample mode"=w105, "samples per channel"=w102, "error in"=w106) -> ("task out"=w104:refnum<k21>, "error out"=w103:errorcluster)  [unwired: 10 in]
            n55 = call <vilib>:"DAQmx Start Task.vi"("task/channels in"=w155, "error in"=w154) -> ("task out"=w126:refnum<k21>, "error out"=w138:errorcluster)  [unwired: 12 in]
            n56 = call <vilib>:"DAQmx Start Task.vi"("task/channels in"=w104, "error in"=w103) -> ("task out"=w111:refnum<k21>, "error out"=w110:errorcluster)  [unwired: 12 in]
            n57 = while {
              tunnel: w130 -> [w201]
              tunnel: w138 -> [w200]
              tunnel: [w199] -> w141
              tunnel: [w198] -> w142
              stop <- w195 stop-if-true
              n58 = call <vilib>:"DAQmx Is Task Done.vi"("task/channels in"=w201, "error in"=w200) -> ("task out"=w199:refnum<k21>, "error out"=w198:errorcluster)  [unwired: 11 in, 1 out]
              n59 = Unbundle By Name(w198) -> ("status"=w197:bool)
              n60 = Or(x=w197, y="stop") -> (x .or. y?=w195:bool)
            }
            n61 = while {
              tunnel: w111 -> [w194]
              tunnel: w110 -> [w193]
              tunnel: [w192] -> w109
              tunnel: [w191] -> w108
              stop <- w188 stop-if-true
              n62 = call <vilib>:"DAQmx Is Task Done.vi"("task/channels in"=w194, "error in"=w193) -> ("task out"=w192:refnum<k21>, "error out"=w191:errorcluster)  [unwired: 11 in, 1 out]
              n63 = Unbundle By Name(w191) -> ("status"=w190:bool)
              n64 = Or(x=w190, y="stop 2") -> (x .or. y?=w188:bool)
            }
            n65 = call <vilib>:"DAQmx Stop Task.vi"("task/channels in"=w141, "error in"=w142) -> ("task out"=w140:refnum<k21>, "error out"=w139:errorcluster)  [unwired: 12 in]
            n66 = call <vilib>:"DAQmx Stop Task.vi"("task/channels in"=w109, "error in"=w108) -> ("task out"=w117:refnum<k21>, "error out"=w118:errorcluster)  [unwired: 12 in]
            n67 = call <vilib>:"DAQmx Clear Task.vi"("task in"=w140, "error in"=w139) -> ("error out"=w125:errorcluster)  [unwired: 13 in]
            n68 = call <vilib>:"DAQmx Clear Task.vi"("task in"=w117, "error in"=w118) -> ("error out"=w116:errorcluster)  [unwired: 13 in]
            n69 = call <vilib>:"DAQmx Stop Task.vi"("task/channels in"=w126, "error in"=w125) -> ("task out"=w143:refnum<k21>, "error out"=w144:errorcluster)  [unwired: 12 in]
            n70 = call <vilib>:"Simple Error Handler.vi"("error in (no error)"=w116) -> ()  [unwired: 4 in, 5 out]
            n71 = call <vilib>:"DAQmx Clear Task.vi"("task in"=w143, "error in"=w144) -> ()  [unwired: 13 in, 1 out]
          }
        }
      }
    }
    frame #3 {
      n72 = invoke class="IAsyncChannel" method="Disable"(reference=w226, error in=w225, "Axis"=w222, "CallType"=u64 0, "pWait"=variant) -> (reference out=w224:refnum<k7>, error out=w223:errorcluster)  [unwired: 1 in, 4 out]
    }
    frame #4 {
      n73 = invoke class="IAsyncChannel" method="CloseComm"(reference=w228, error in=w227) -> (error out=→"Error out":errorcluster)  [unwired: 1 in, 2 out]
    }
    frame #5 {
      n74 = local write "Connected"(FALSE ("Connected")) -> ()
    }
  }
